vi "max_min_error_v00.vi"(8 "Array":dbl[](array[numeric]), 10 "maxmin":bool) -> (0 "max value":dbl, 1 "x+y":dbl(slide) scale=0.0..10.0, 2 "min value":dbl)   [LabVIEW 2013]
doc: "Calculates running average. (Needs tidying)."
uses:
  <vilib>/express/express arith-compare/Formula/XNode/ExpressFormulaBlockNode.xnode
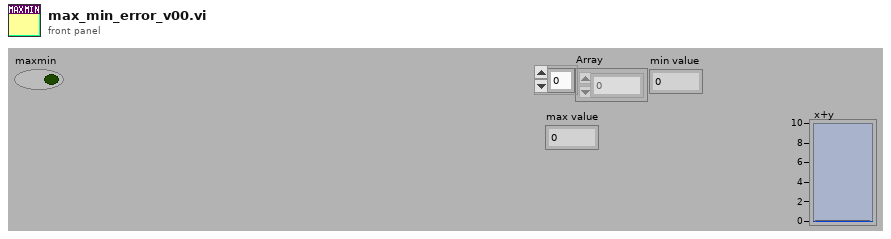
[diagram p1: front panel]
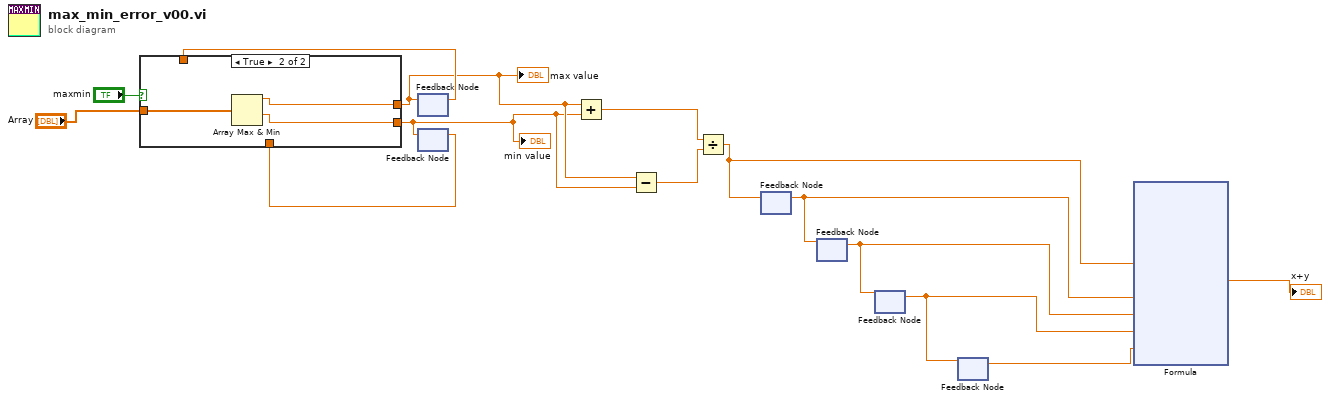
[diagram p0: block diagram]
diagram:
  n1 = feedback #1() -> (w12:dbl)  [unwired: 1 in]
  n2 = feedback #2() -> (w11:dbl)  [unwired: 1 in]
  n3 = case shown="True" "maxmin" {
    tunnel: "Array" -> [_ w19]
    tunnel: [w16 w18] -> w10
    tunnel: [w15 w17] -> w9
    tunnel: w12 -> [w16 _]
    tunnel: w11 -> [w15 _]
    frame False {
    }
    frame True {
      n4 = Array Max & Min(array=w19) -> (max value=w18:dbl, min value=w17:dbl)  [unwired: 2 out]
    }
  }
  "max value" <- w10
  "min value" <- w9
  n5 = feedback-in #1(w10) -> ()
  n6 = feedback-in #2(w9) -> ()
  n7 = Add(x=w10, y=w9) -> (x+y=w8:dbl)
  n8 = Subtract(x=w10, y=w9) -> (x-y=w7:dbl)
  n9 = Divide(x=w8, y=w7) -> (x/y=w6:dbl)
  n10 = feedback #3() -> (w5:dbl)  [unwired: 1 in]
  n11 = feedback-in #3(w6) -> ()
  n12 = feedback #4() -> (w4:dbl)  [unwired: 1 in]
  n13 = feedback-in #4(w5) -> ()
  n14 = feedback #5() -> (w3:dbl)  [unwired: 1 in]
  n15 = feedback-in #5(w4) -> ()
  n16 = feedback #6() -> (w2:dbl)  [unwired: 1 in]
  n17 = feedback-in #6(w3) -> ()
  n18 = xnode "Formula"("X1"=w6, "X2"=w5, "X3"=w4, "X4"=w3, "X5"=w2) -> ("Result"=→"x+y":dbl)  [unwired: 1 in, 1 out]
